vi "Ball Screw Control.vi"(2 "Target Button":bool, 7 "Joystick Axis":dbl, 8 "Bot Limit":bool, 9 "Top Limit":bool, 10 "Closed Loop On/Off":bool, 11 "Ball Screw DevRef In":T1={"DeviceStatus"={"status"=FALSE, "code"=0, "source"=""}, "Type"=enum."PWM", "PWM"={"Digital Module"=enum."Digital Module 1", "PWM Channel"=enum."Invalid", "DeadBand"={"Name"="", "maxPositivePwm"=0, "minPositivePwm"=0, "centerPwm"=0, "maxNegativePwm"=0, "minNegativePwm"=0, "angularRange"=0}}, "CAN"={"Device Number"=0, "Control Mode"=enum."Percent VBus", "Semaphore"=refnum, "Max Vout"=12.0}, "Invert"=FALSE, "TransformRef"=refnum, "InvTransformRef"=refnum}) -> (1 "Motor Output":dbl, 3 "Ball Screw DevRef Out":T1={"DeviceStatus"={"status"=FALSE, "code"=0, "source"=""}, "Type"=enum."PWM", "PWM"={"Digital Module"=enum."Digital Module 1", "PWM Channel"=enum."Invalid", "DeadBand"={"Name"="", "maxPositivePwm"=0, "minPositivePwm"=0, "centerPwm"=0, "maxNegativePwm"=0, "minNegativePwm"=0, "angularRange"=0}}, "CAN"={"Device Number"=0, "Control Mode"=enum."Percent VBus", "Semaphore"=refnum, "Max Vout"=12.0}, "Invert"=FALSE, "TransformRef"=refnum, "InvTransformRef"=refnum})   [LabVIEW 2012]
uses:
  <vilib>/Rock Robotics/WPI/MotorControl/WPI_MotorControlDeviceRef.ctl
  <vilib>/Rock Robotics/SystemInterfaces/Typedef/FPGA_TypedefDigitalModule.ctl
  <vilib>/Rock Robotics/SystemInterfaces/DIO/FPGA_DIOPWMChannel.ctl
  <vilib>/Rock Robotics/WPI/PWM/WPI_PWMDeadband.ctl
  <vilib>/Rock Robotics/WPI/CAN/Jaguar/SubVIs/WPI_CANJaguar_ControlMode.ctl
  <vilib>/Rock Robotics/WPI/PWM/WPI_PWMTransform_ConPane.ctl
  <vilib>/Rock Robotics/WPI/CAN/Jaguar/SubVIs/WPI_CANJaguar_PositionReference.ctl
  Robot Global Data.vi
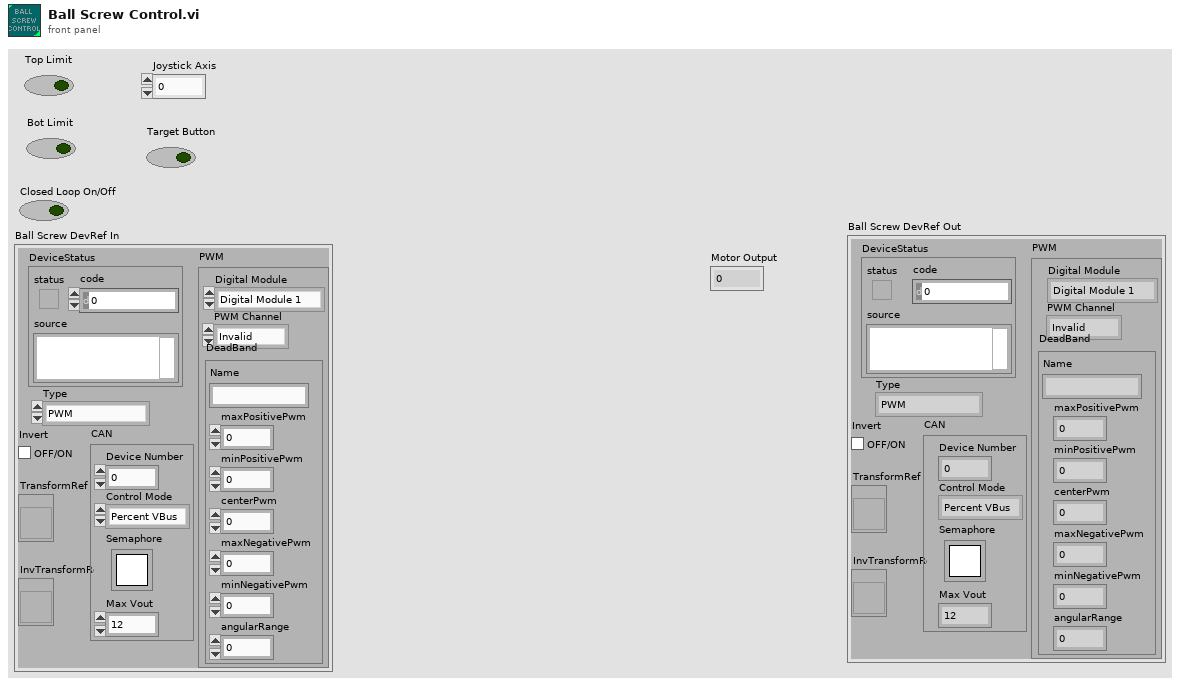
[diagram p1: front panel]
types:
  T1 = typedef "WPI_MotorControlDeviceRef.ctl" = cluster{"DeviceStatus":errorcluster, "Type":enum16{"PWM", "CAN"}, "PWM":cluster{"Digital Module":T2, "PWM Channel":T3, "DeadBand":T4}, "CAN":cluster{"Device Number":u8, "Control Mode":T5, "Semaphore":T6, "Max Vout":dbl}, "Invert":bool, "TransformRef":T7, "InvTransformRef":T7}
  T2 = typedef "FPGA_TypedefDigitalModule.ctl" = enum16{"Digital Module 1", "Digital Module 2"}
  T3 = typedef "FPGA_DIOPWMChannel.ctl" = enum8{"PWM 1", "PWM 2", "PWM 3", "PWM 4", "PWM 5", "PWM 6", "PWM 7", "PWM 8", "PWM 9", "PWM 10", "Invalid"}
  T4 = typedef "WPI_PWMDeadband.ctl" = cluster{"Name":string, "maxPositivePwm":i32, "minPositivePwm":i32, "centerPwm":i32, "maxNegativePwm":i32, "minNegativePwm":i32, "angularRange":u16}
  T5 = typedef "WPI_CANJaguar_ControlMode.ctl" = enum8{"Percent VBus", "Current", "Speed", "Position", "Voltage"}
  T6 = typedef "Semaphore RefNum" = refnum<k1>
  T7 = typedef "WPI_PWMTransform_ConPane.ctl" = refnum<vi>
  T8 = typedef "WPI_CANJaguar_PositionReference.ctl" = u8
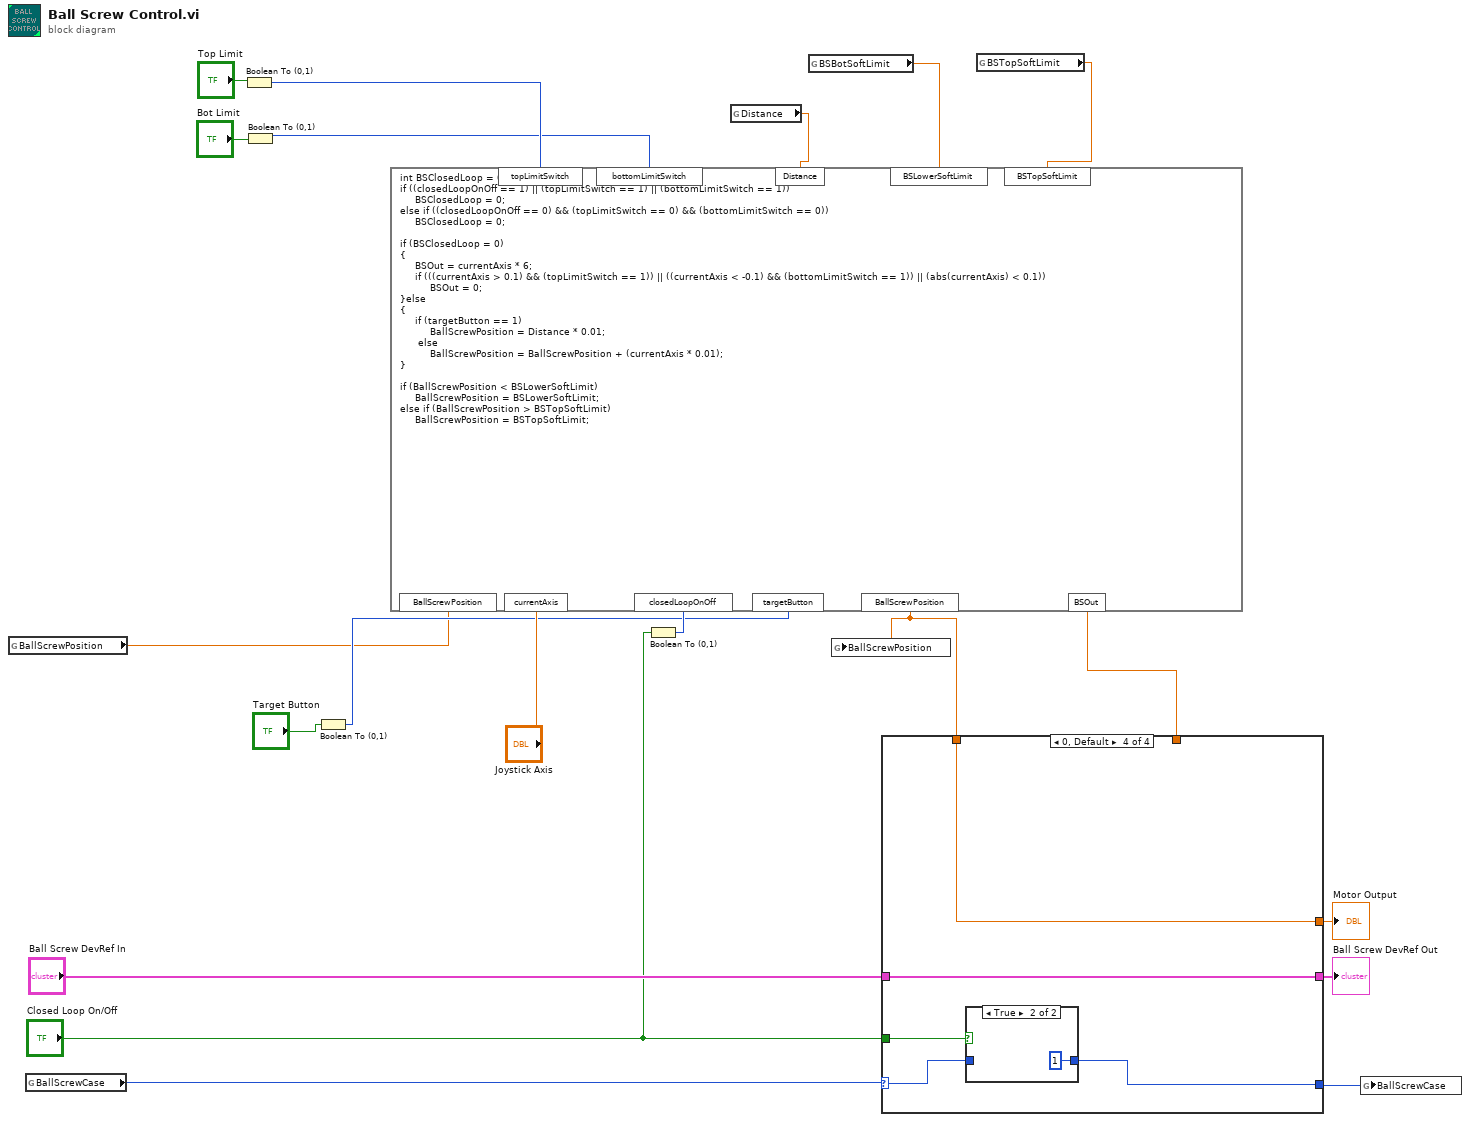
[diagram p0: block diagram]
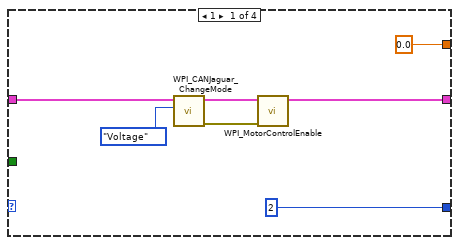
[diagram p2: hidden frame]
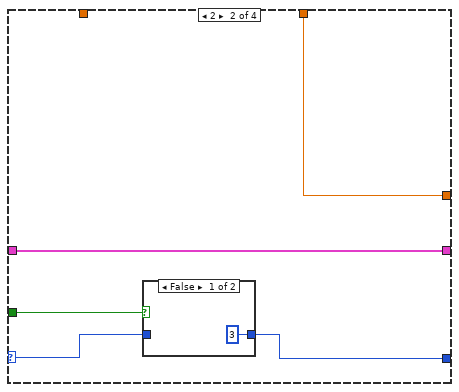
[diagram p3: hidden frame]
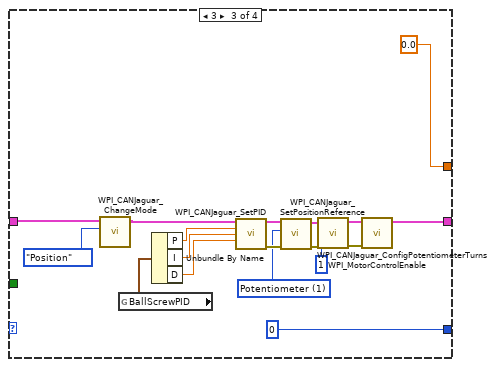
[diagram p5: hidden frame]
diagram:
  n1 = global read "Robot Global Data.vi" "BallScrewPosition"() -> (w8:dbl)
  n2 = global read "Robot Global Data.vi" "BallScrewCase"() -> (w20:i8)
  n3 = Boolean To (0,1)(Boolean="Top Limit") -> (0, 1=w14:i16)
  n4 = Boolean To (0,1)(Boolean="Bot Limit") -> (0, 1=w13:i16)
  n5 = Boolean To (0,1)(Boolean="Target Button") -> (0, 1=w9:i16)
  n6 = Boolean To (0,1)(Boolean="Closed Loop On/Off") -> (0, 1=w17:i16)
  n7 = global read "Robot Global Data.vi" "Distance"() -> (w7:dbl)
  n8 = global read "Robot Global Data.vi" "BSBotSoftLimit"() -> (w6:dbl)
  n9 = global read "Robot Global Data.vi" "BSTopSoftLimit"() -> (w5:dbl)
  n10 = formula code="int BSClosedLoop = 0;\nif ((closedLoopOnOff == 1) || (topLimitSwitch == 1) || (bottomLimitSwitch == 1))\n     BSClosedLoop = 0;\nelse if ((closedLoopOnOff == 0) && (topLimitSwitch == 0) && (bottomLimitSwitch == 0))\n     BSClosedLoop = 0;\n\nif (BSClosedLoop = 0)\n{\n     BSOut = currentAxis * 6;\n     if (((currentAxis > 0.1) && (topLimitSwitch == 1)) || ((currentAxis < -0.1) && (bottomLimitSwitch == 1)) || (abs(currentAxis) < 0.1))\n          BSOut = 0;\n}else\n{\n     if (targetButton == 1)\n          BallScrewPosition = Distance * 0.01;\n      else\n          BallScrewPosition = BallScrewPosition + (currentAxis * 0.01);\n}\n\nif (BallScrewPosition < BSLowerSoftLimit)\n     BallScrewPosition = BSLowerSoftLimit;\nelse if (BallScrewPosition > BSTopSoftLimit)\n     BallScrewPosition = BSTopSoftLimit;"("closedLoopOnOff"=w17, "topLimitSwitch"=w14, "bottomLimitSwitch"=w13, "BallScrewPosition"=w8, "currentAxis"="Joystick Axis", "targetButton"=w9, "Distance"=w7, "BSLowerSoftLimit"=w6, "BSTopSoftLimit"=w5) -> ("BSOut"=w11:dbl, "BallScrewPosition"=w4:dbl)
  n11 = global write "Robot Global Data.vi" "BallScrewPosition"(w4) -> ()
  n12 = case shown="0, Default" w20 {
    selector: w20 -> [_ w30 _ w54]
    tunnel: [i8 2 ("ShooterCase") w29 i8 0 ("ShooterCase") w55] -> w1
    tunnel: "Ball Screw DevRef In" -> [w26 w32 w51 w57]
    tunnel: [w22 w32 w38 w57] -> w2
    tunnel: "Closed Loop On/Off" -> [_ w31 _ w56]
    tunnel: [0.0 ("FSpeed") w28 0.0 ("FSpeed") w53] -> w3
    tunnel: w11 -> [_ w28 _ _]
    tunnel: w4 -> [_ _ _ w53]
    frame 1 {
      n13 = call <vilib>:"WPI_CANJaguar_ChangeMode.vi"("Control Mode"=WPI_CANJaguar_ControlMode."Voltage", "CAN Jaguar Ref"=w26) -> ("error out"=w23:errorcluster, "CAN Jaguar Ref Out"=w24:T1)  [unwired: 8 in]
      n14 = call <vilib>:"WPI_MotorControlEnable.vi"("error in (no error)"=w23, "CAN Jaguar Ref"=w24) -> ("CAN Jaguar Ref Out"=w22:T1)  [unwired: 8 in, 1 out]
    }
    frame 2 {
      n15 = case shown="False" w31 {
        tunnel: [i8 3 ("ShooterCase") w34] -> w29
        tunnel: w30 -> [_ w34]
        frame False {
        }
        frame True {
        }
      }
    }
    frame 3 {
      w36 = T8 1 items=["Quad Encoder"=0, "Potentiometer"=1, "None"=255] ("Position Reference")
      n16 = call <vilib>:"WPI_CANJaguar_ChangeMode.vi"("Control Mode"=WPI_CANJaguar_ControlMode."Position", "CAN Jaguar Ref"=w51) -> ("CAN Jaguar Ref Out"=w46:T1)  [unwired: 8 in, 1 out]
      n17 = global read "Robot Global Data.vi" "BallScrewPID"() -> (w50:cluster{"P":dbl, "I":dbl, "D":dbl})
      n18 = Unbundle By Name(w50) -> ("P"=w49:dbl, "I"=w48:dbl, "D"=w47:dbl)
      n19 = call <vilib>:"WPI_CANJaguar_SetPID.vi"("CAN Jaguar Ref"=w46, "P"=w49, "I"=w48, "D"=w47) -> ("CAN Jaguar Ref Out"=w44:T1, "error out"=w43:errorcluster)  [unwired: 10 in]
      n20 = call <vilib>:"WPI_CANJaguar_SetPositionReference.vi"("error in (no error)"=w43, "Position Reference"=w36, "CAN Jaguar Ref"=w44) -> ("error out"=w41:errorcluster, "CAN Jaguar Ref Out"=w42:T1)  [unwired: 7 in]
      n21 = call <vilib>:"WPI_CANJaguar_ConfigPotentiometerTurns.vi"("error in (no error)"=w41, "Potentiometer Turns"=u16 1, "CAN Jaguar Ref"=w42) -> ("error out"=w40:errorcluster, "CAN Jaguar Ref Out"=w39:T1)  [unwired: 7 in]
      n22 = call <vilib>:"WPI_MotorControlEnable.vi"("error in (no error)"=w40, "CAN Jaguar Ref"=w39) -> ("CAN Jaguar Ref Out"=w38:T1)  [unwired: 8 in, 1 out]
    }
    frame 0, Default {
      n23 = case shown="True" w56 {
        tunnel: [w58 i8 1 ("ShooterCase")] -> w55
        tunnel: w54 -> [w58 _]
        frame False {
        }
        frame True {
        }
      }
    }
  }
  "Motor Output" <- w3
  "Ball Screw DevRef Out" <- w2
  n24 = global write "Robot Global Data.vi" "BallScrewCase"(w1) -> ()
